vi "Do.vi"(8 "error in (no error)":errorcluster, 10 "Actor in":refnum<class "Actor.lvclass">, 11 "Process New Connection Request Msg":refnum<class "Process Connection Msg.lvclass">) -> (0 "error out":errorcluster, 2 "Actor out":refnum<class "Actor.lvclass">)   [LabVIEW 2019, in "ConnectionFactorySession.lvlib" / "Process Connection Msg.lvclass"]
doc: "This VI delivers the message to the actor by calling the appropriate method(s) on the actor."
uses:
  <vilib>/gpm_packages/@cs/Network-interface/Source/Connection Factory Session/Messages/Process Connection Msg/Process Connection Msg.lvclass
  <vilib>/ActorFramework/Actor/Actor.lvclass
  <vilib>/gpm_packages/@cs/Network-interface/Source/Connection Factory Session/ConnectionFactoryHandler/ConnectionFactoryHandler.lvclass
  C:/Program Files/National Instruments/LabVIEW 2019/vi.lib/gpm_packages/@cs/Network-interface/Source/Logged Actor/LoggedActor.lvclass
  C:/Program Files/National Instruments/LabVIEW 2019/vi.lib/ActorFramework/Actor/Actor.lvclass
  <vilib>/gpm_packages/@cs/Network-interface/Source/Connection Factory Session/Messages/Process Connection Msg/Process Connection Msg.lvclass/Process Connection Msg.ctl
  <vilib>/gpm_packages/@cs/Network-interface/Source/Logged Actor/LoggedActor.lvclass/LoggedActor.ctl
  <vilib>/gpm_packages/@cs/event-logger/Source/Composed Log/LoggerReference/LoggerReference.lvclass/LoggerReference.ctl
  <vilib>/gpm_packages/@cs/Network-interface/Source/Connection Factory Session/ConnectionFactoryHandler/ConnectionFactoryHandler.lvclass/ConnectionFactoryHandler.ctl
  <vilib>/ActorFramework/Actor/Actor.lvclass/Actor.ctl
  <vilib>/ActorFramework/Message Enqueuer/Message Enqueuer.lvclass/Message Enqueuer.ctl
  <vilib>/gpm_packages/@cs/Network-interface/Source/Connection Factory Session/ConnectionFactoryHandler/Create Connection.vi
  <vilib>/gpm_packages/@cs/Network-interface/Source/Logged Actor/Log Session Event.vi
  <vilib>/gpm_packages/@cs/Network-interface/Source/Connection Factory Session/Messages/Create Connection Msg/Send Create Connection.vi
  <vilib>/ActorFramework/Actor/Read Self Enqueuer.vi
  <vilib>/gpm_packages/@cs/Network-interface/Source/Connection Factory Session/ConnectionFactoryHandler/Update Connection Cache.vi
  <vilib>/gpm_packages/@cs/event-logger/Source/Composed Log/LoggerReference/Log Event.vi
  <vilib>/ActorFramework/Message Enqueuer/Enqueue.vi
  <vilib>/ActorFramework/Message Enqueuer/Init from Existing Queue.vi
  <vilib>/gpm_packages/@cs/event-logger/Source/Composed Log/LoggerReference/Log.vi
  <vilib>/gpm_packages/@cs/event-logger/Source/Composed Log/LoggerReference/Get Valid Event Time.vi
  <vilib>/gpm_packages/@cs/event-logger/Source/Composed Log/LoggerReference/Remove Stale Logs.vi
  <vilib>/gpm_packages/@cs/Network-interface/Source/Connection Factory Session/Messages/Create Connection Msg/Create Connection Msg.lvclass
  C:/Program Files/National Instruments/LabVIEW 2019/vi.lib/ActorFramework/Message/Message.lvclass
  <vilib>/gpm_packages/@cs/Network-interface/Source/Connection Reference/Connection Reference/Construct Connection Reference.vi
  <vilib>/gpm_packages/@cs/Network-interface/Source/Connection Reference/Connection Reference/Close Connection.vi
  <vilib>/ActorFramework/Message Priority Queue/Priority Enqueue.vi
  <vilib>/gpm_packages/@cs/Network-interface/Source/Connection Reference/IConnection/IConnection.lvclass
  <vilib>/gpm_packages/@cs/Network-interface/Source/Connection Reference/Connection Reference/Connection Reference.lvclass
  <vilib>/ActorFramework/Message Enqueuer/Message Enqueuer.lvclass
  <vilib>/gpm_packages/@cs/Network-interface/Source/IConnectionFactory/IConnectionFactory.lvclass
  <vilib>/gpm_packages/@cs/Network-interface/Source/Connection Factory Session/INewConnectionCallback/INewConnectionCallback.lvclass
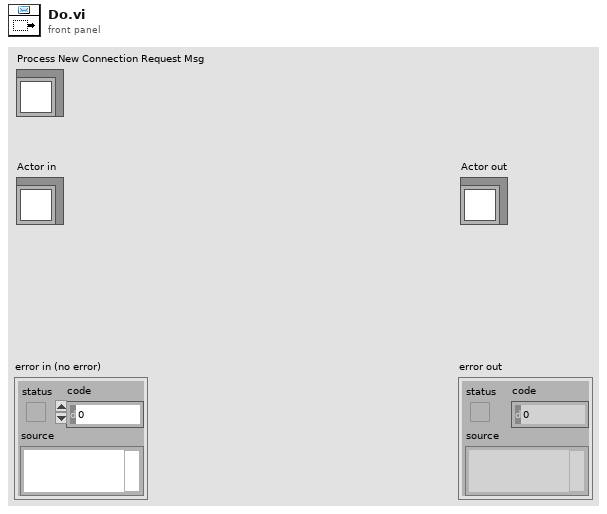
[diagram p1: front panel]
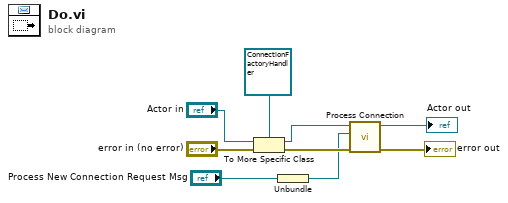
[diagram p0: block diagram]
diagram:
  n1 = To More Specific Class(target class=refnum<class "ConnectionFactoryHandler.lvclass"> refnum ("Actor in"), reference="Actor in", error in="error in (no error)") -> (specific class reference=w1:refnum<class "ConnectionFactoryHandler.lvclass">, error out=w7:errorcluster)
  n2 = Unbundle("Process New Connection Request Msg") -> (w2:refnum<class "INewConnectionCallback.lvclass">)
  n3 = call <vilib>:"Process Connection.vi"("error in (no error)"=w7, "New Connection Policy"=w2, "ConnectionFactoryHandler in"=w1) -> ("error out"=→"error out":errorcluster, "ConnectionFactoryHandler out"=→"Actor out":refnum<class "ConnectionFactoryHandler.lvclass">)  [unwired: 7 in]
